vi "Sim Configurations.vi"(8 "error constant":errorcluster, 10 "Base Station":T4, 11 "Cluster in":T1) -> (0 "error constant":errorcluster, 3 "Cluster out":T1)   [LabVIEW 2021]
uses:
  APIs/Controls/Base_Station_Emulator.ctl
  IP Simulation/Controls/Enum-TypeDef.ctl
  Save File/Sim_Confi.ctl
panel:
  out "Data Out":T2
  in  "Enum":T3
  in  "SIM_U_Config":T2
  # "IMSI"
  # "TAC"
  # "K Value"
  # "OP Value"
  # "Edit"
  # "Actions"
  # "Phone Number"
  # "Sim Configurations"
  # "ASDFADFAF"
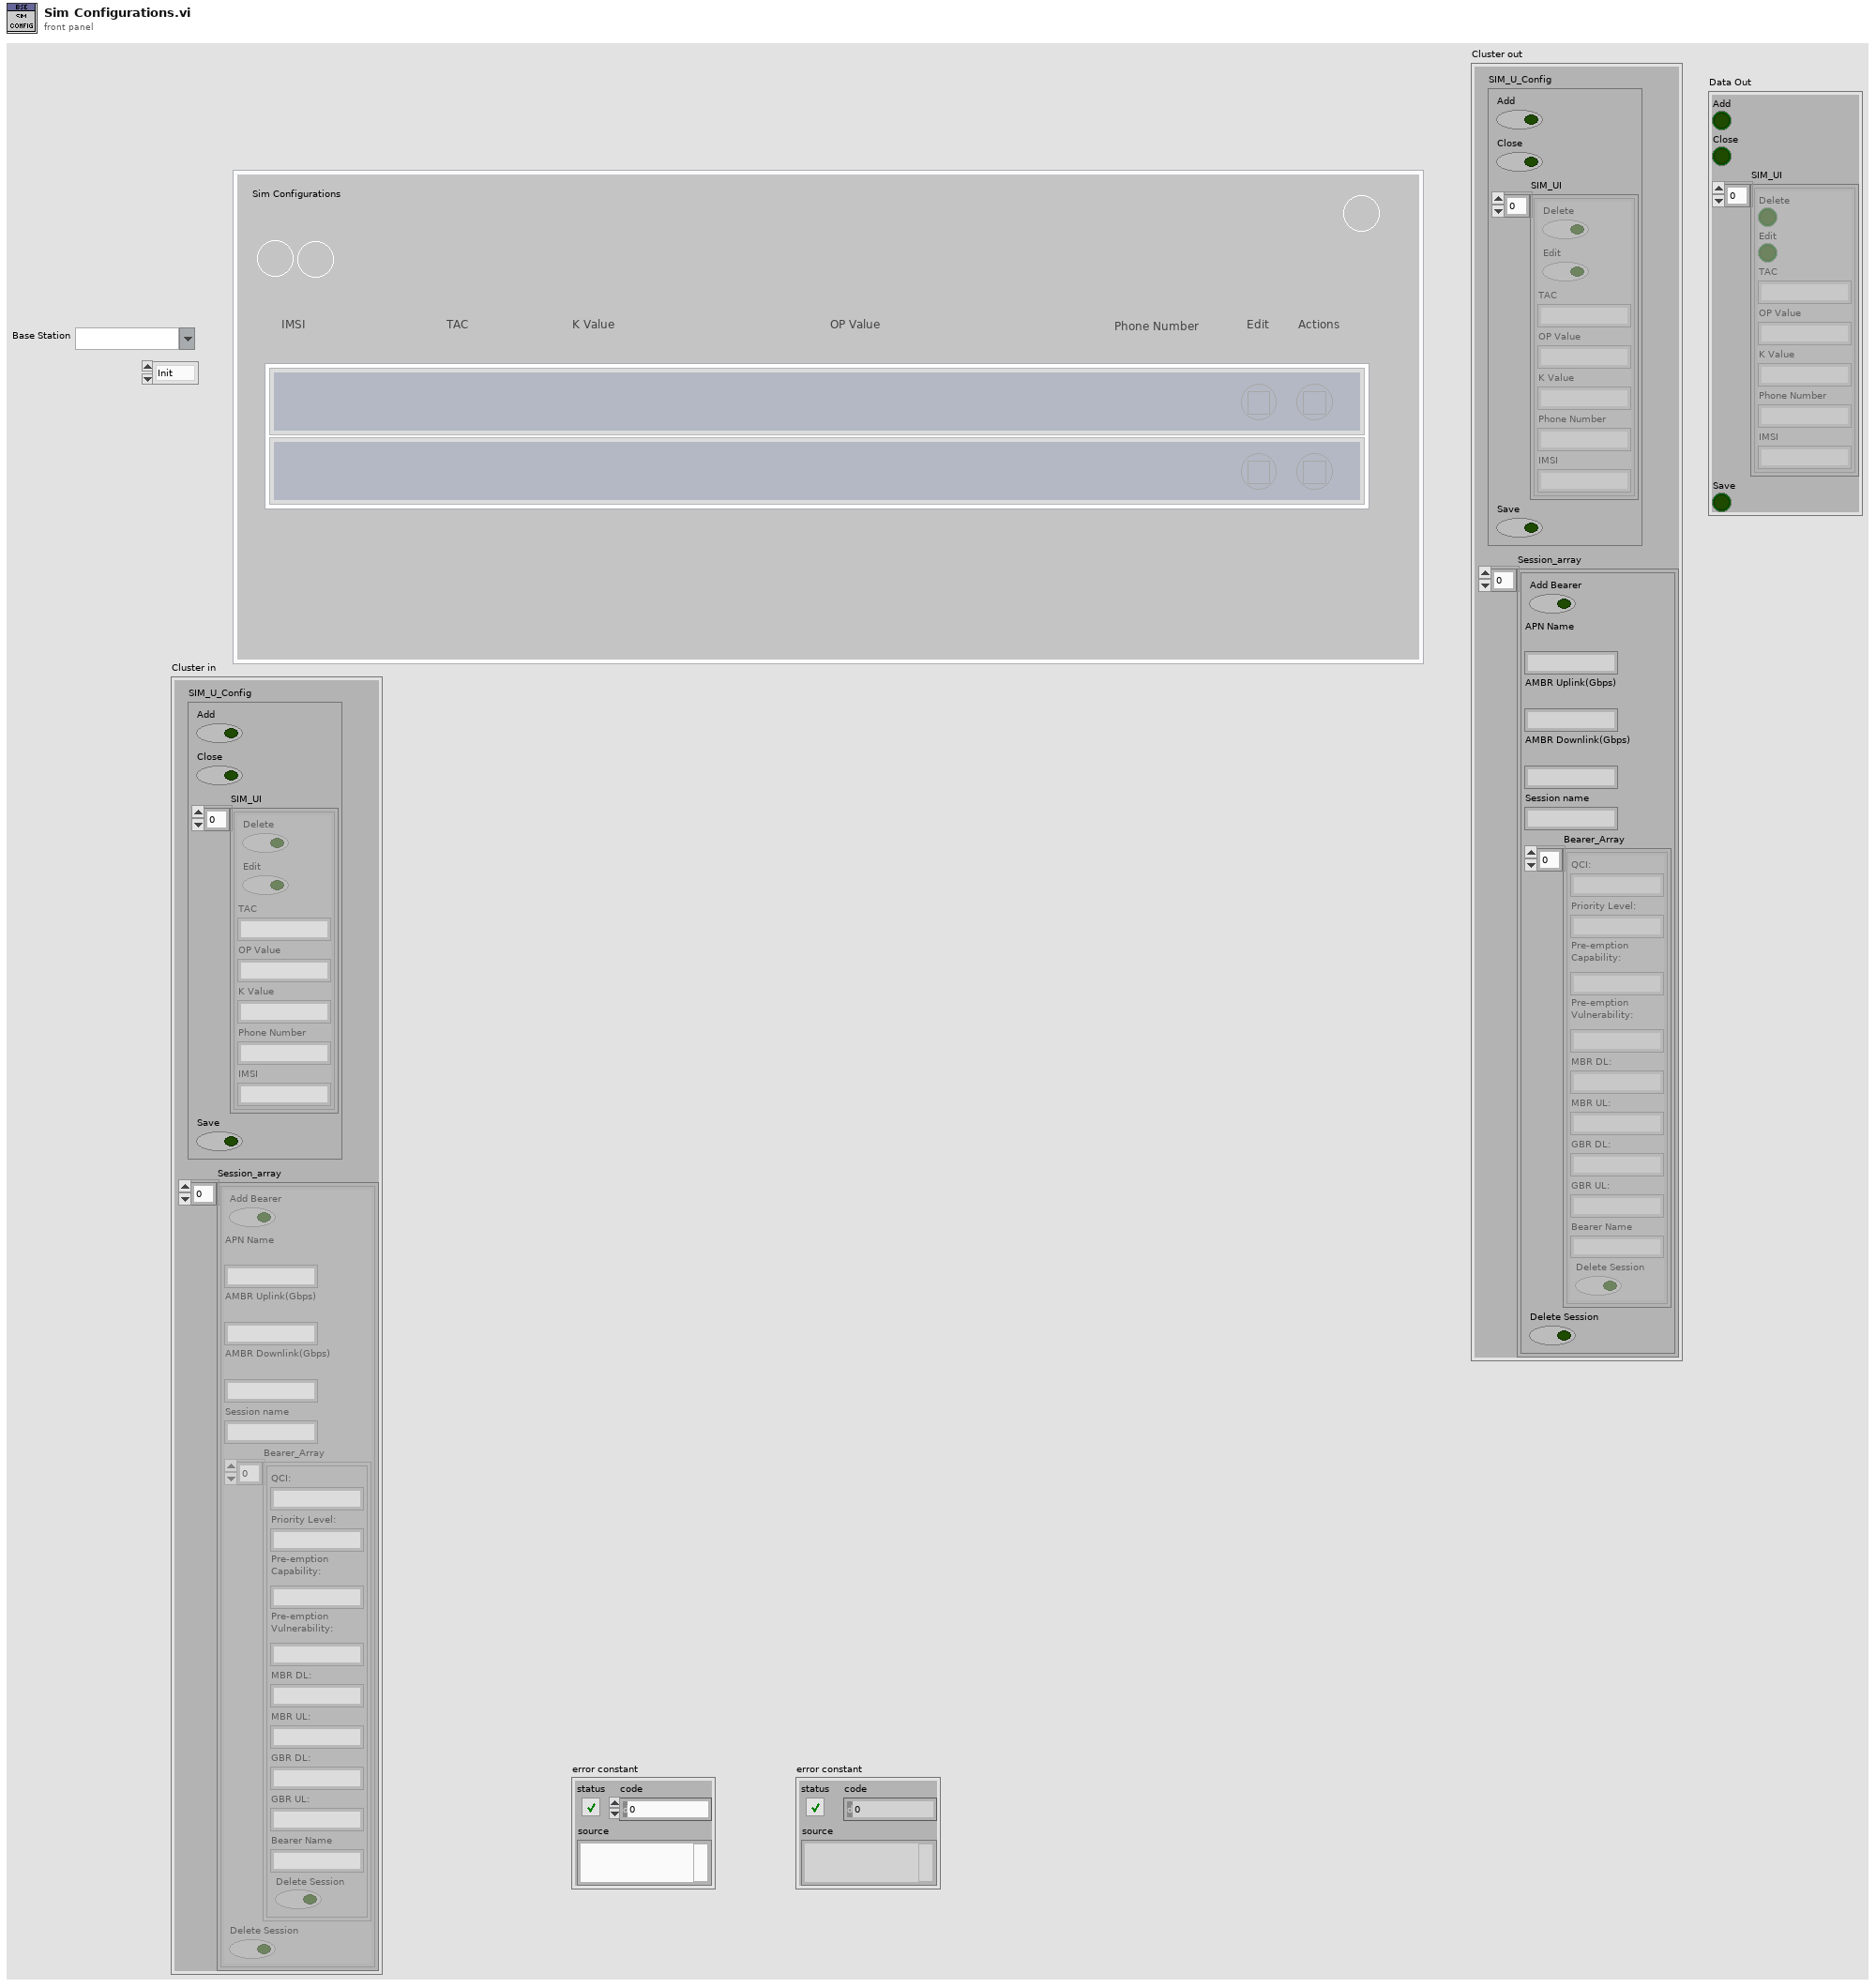
[diagram p1: front panel]
types:
  T1 = typedef "Sim_Confi.ctl" = cluster{"Session_array":cluster{"Add Bearer":bool, "APN Name\n":string, "AMBR Uplink(Gbps)\n":string, "AMBR Downlink(Gbps)\n":string, "Session name":string, "Bearer_Array":cluster{"QCI:":string, "Priority Level:":string, "Pre-emption\nCapability:":string, "Pre-emption\nVulnerability:":string, "MBR DL:":string, "MBR UL:":string, "GBR DL:":string, "GBR UL:":string, "Bearer Name":string, "Delete Session":bool}[], "Delete Session":bool}[], "SIM_U_Config":cluster{"Add":bool, "Close":bool, "SIM_UI":cluster{"Delete":bool, "Edit":bool, "TAC":string, "OP Value":string, "K Value":string, "Phone Number":string, "IMSI":string}[], "Save":bool}}
  T2 = cluster{"Add":bool, "Close":bool, "SIM_UI":cluster{"Delete":bool, "Edit":bool, "TAC":string, "OP Value":string, "K Value":string, "Phone Number":string, "IMSI":string}[], "Save":bool}
  T3 = typedef "Enum-TypeDef.ctl" = enum16{"Init", "poll", "Close"}
  T4 = typedef "Base_Station_Emulator.ctl" = string
  T5 = cluster{"Delete":bool, "Edit":bool, "TAC":string, "OP Value":string, "K Value":string, "Phone Number":string, "IMSI":string}[]
  T6 = cluster{"Add Bearer":bool, "APN Name\n":string, "AMBR Uplink(Gbps)\n":string, "AMBR Downlink(Gbps)\n":string, "Session name":string, "Bearer_Array":cluster{"QCI:":string, "Priority Level:":string, "Pre-emption\nCapability:":string, "Pre-emption\nVulnerability:":string, "MBR DL:":string, "MBR UL:":string, "GBR DL:":string, "GBR UL:":string, "Bearer Name":string, "Delete Session":bool}[], "Delete Session":bool}[]
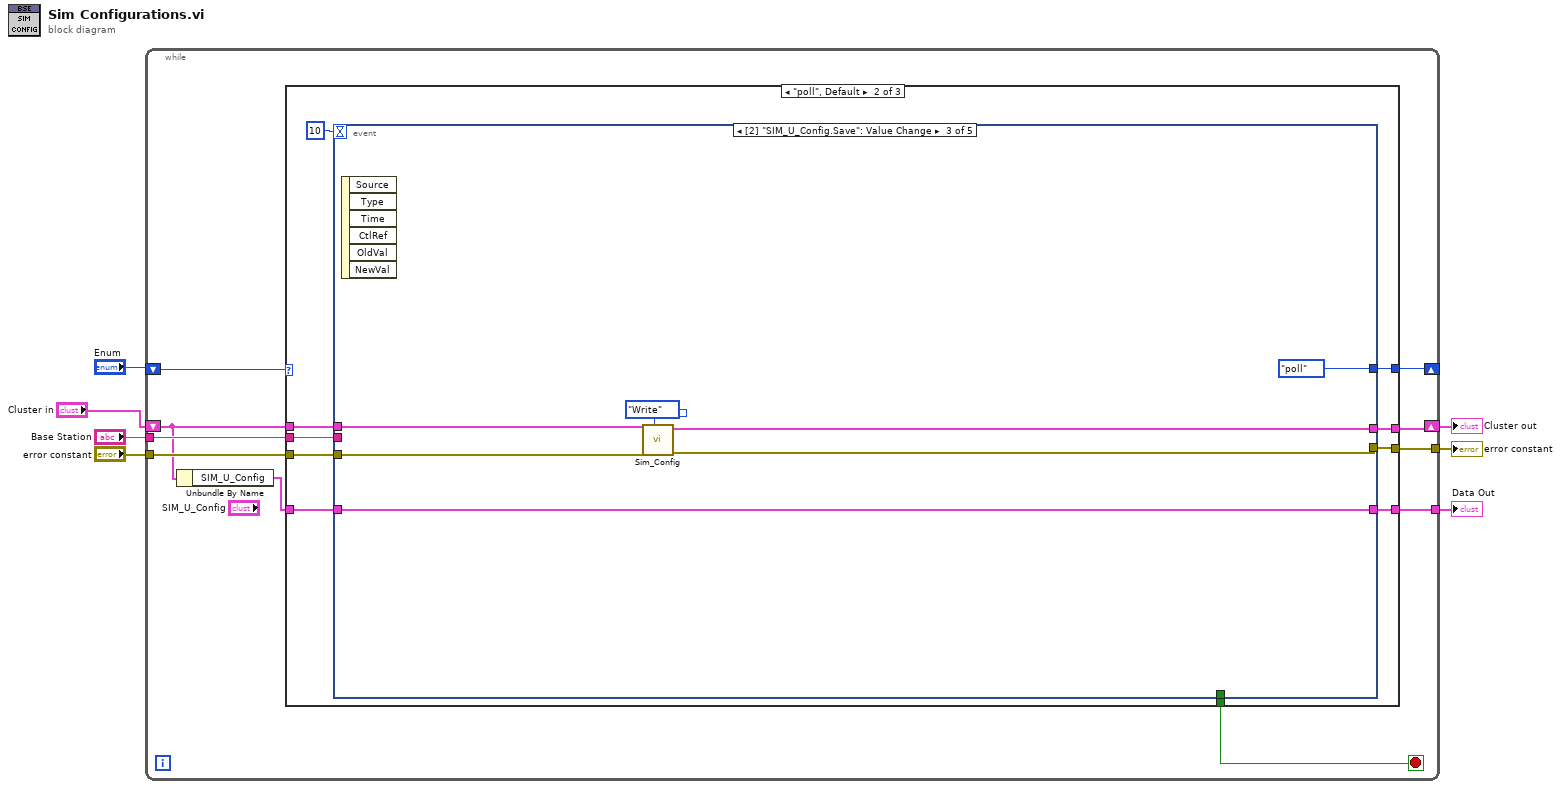
[diagram p0: block diagram]
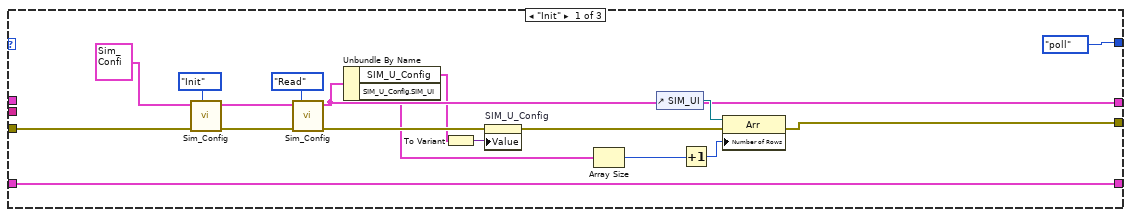
[diagram p2: hidden frame]
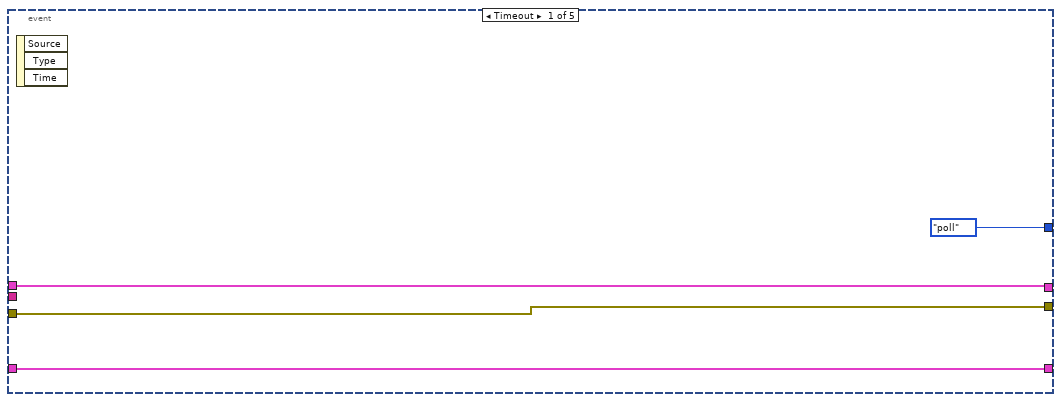
[diagram p3: hidden frame]
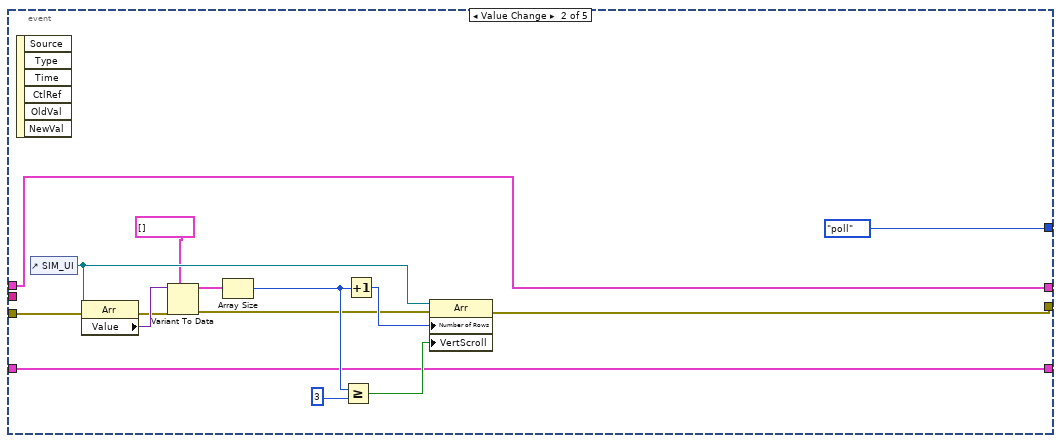
[diagram p4: hidden frame]
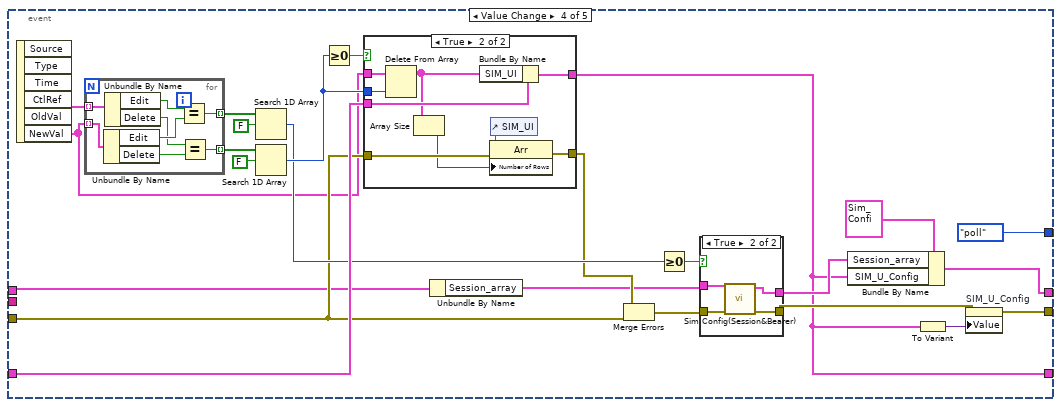
[diagram p5: hidden frame]
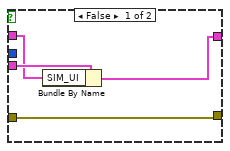
[diagram p6: hidden frame]
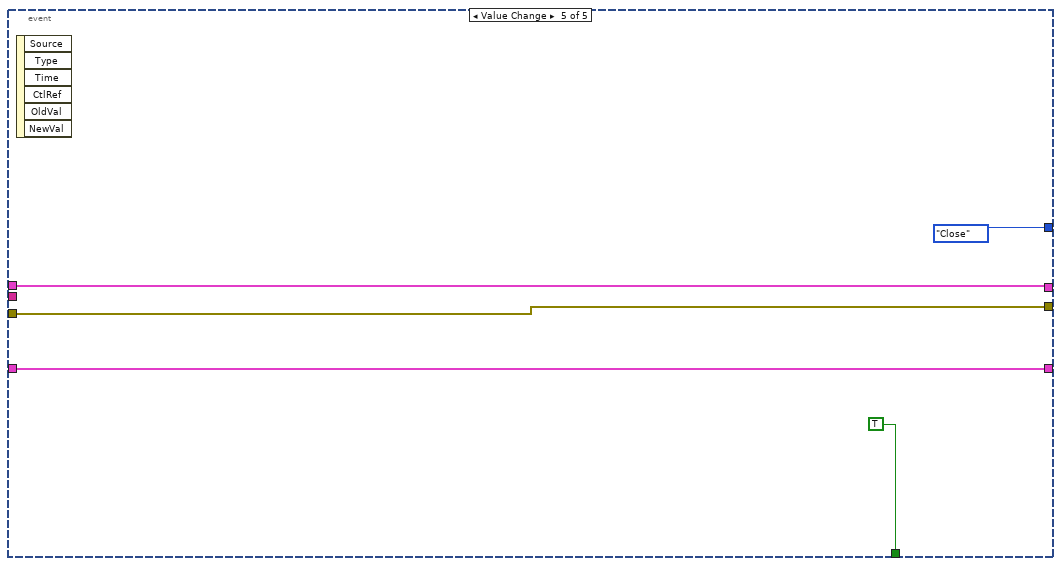
[diagram p8: hidden frame]
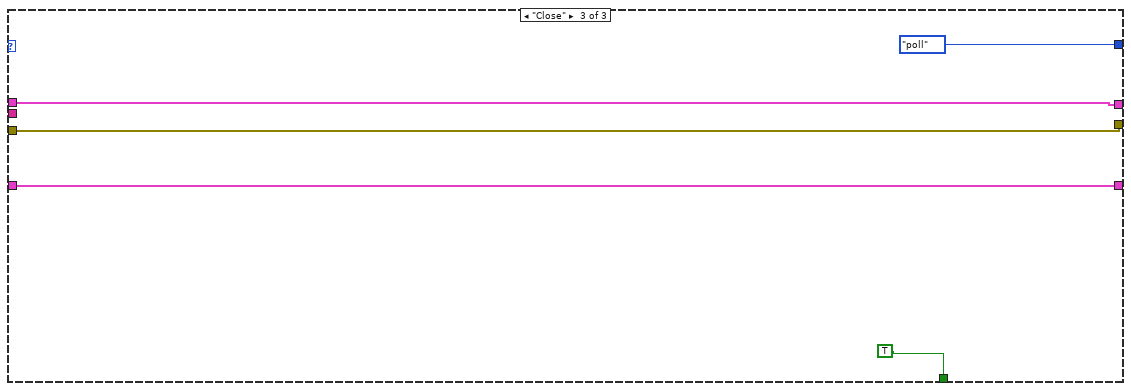
[diagram p9: hidden frame]
diagram:
  n1 = while {
    shift-right: [w15] -> _
    shift-left: "Enum" -> [w16]
    tunnel: "error constant" -> [w14]
    tunnel: [w13] -> w4
    tunnel: "Base Station" -> [w12]
    tunnel: [w11] -> w3
    shift-right: [w10] -> w2
    shift-left: "Cluster in" -> [w9]
    stop <- w17 stop-if-true
    n2 = Unbundle By Name(w9) -> ("SIM_U_Config"=w8:T2)
    n3 = case shown="\"poll\", Default" w16 {
      tunnel: [_ w38 TRUE] -> w17
      tunnel: [Enum-TypeDef."poll" w43 Enum-TypeDef."poll"] -> w15
      tunnel: w14 -> [w21 w45 w131]
      tunnel: [w19 w44 w131] -> w13
      tunnel: w8 -> [w27 w41 w129]
      tunnel: w12 -> [_ w40 _]
      tunnel: [w27 w39 w129] -> w11
      tunnel: [w26 w37 w128] -> w10
      tunnel: w9 -> [_ w36 w128]
      frame "Init" {
        n4 = call "Sim_Config.vi"("Hardware Case Selection"=enum16{"Init", "Read", "Write", "Close"}."Init", "error in (no error)"=w21, 11:T1 {"Session_array"=[{"Add Bearer"=FALSE, "APN Name\n"="", "AMBR Uplink(Gbps)\n"="", "AMBR Downlink(Gbps)\n"="", "Session name"="", "Bearer_Array"=[], "Delete Session"=FALSE}], "SIM_U_Config"={"Add"=FALSE, "Close"=FALSE, "SIM_UI"=[], "Save"=FALSE}}) -> ("error out"=w30:errorcluster, "Cluster"=w22:T1)  [unwired: 7 in]
        n5 = call "Sim_Config.vi"("Hardware Case Selection"=enum16{"Init", "Read", "Write", "Close"}."Read", "error in (no error)"=w30, 11:w22) -> ("error out"=w28:errorcluster, "Cluster"=w26:T1)  [unwired: 7 in]
        n6 = Unbundle By Name(w26) -> ("SIM_U_Config"=w24:T2, "SIM_U_Config.SIM_UI"=w18:T5)
        n7 = To Variant(anything=w24) -> (Variant=w25:variant)
        n8 = property on="SIM_U_Config" class="Clust"(error in=w28, "Value"=w25) -> (error out=w20:errorcluster)  [unwired: 1 in, 1 out]
        n9 = Array Size(array=w18) -> (size(s)=w33:i32)
        n10 = control-ref of="SIM_UI"() -> (w34:refnum<vi>)
        n11 = Increment(x=w33) -> (x+1=w32:i32)
        n12 = property class="Arr"(reference=w34, error in=w20, "Number of Rows"=w32) -> (error out=w19:errorcluster)  [unwired: 1 out]
      }
      frame "poll", Default {
        n13 = event shown="[2] \"SIM_U_Config.Save\": Value Change" {
          selector: _ -> [_ _ _ _ _]
          dyn-events: _ -> [_ _ _ _ _]
          timeout: 10 -> [_ _ _ _ _]
          tunnel: w45 -> [w47 w53 w69 w82 w126]
          tunnel: [w47 w60 w68 w86 w126] -> w44
          tunnel: [Enum-TypeDef."poll" Enum-TypeDef."poll" Enum-TypeDef."poll" Enum-TypeDef."poll" Enum-TypeDef."Close"] -> w43
          tunnel: w40 -> [_ _ _ _ _]
          tunnel: w41 -> [w48 w55 w66 w85 w125]
          tunnel: [w48 w55 w66 w72 w125] -> w39
          tunnel: [_ _ _ _ TRUE] -> w38
          tunnel: [w46 w50 w65 w78 w123] -> w37
          tunnel: w36 -> [w46 w50 w70 w77 w123]
          event Timeout {
            n14 = event-data() -> ()  [unwired: 1 in, 3 out]
          }
          event "SIM_U_Config.Add": Value Change {
            n15 = event-data() -> ()  [unwired: 1 in, 6 out]
            n16 = control-ref of="SIM_UI"() -> (w58:refnum<vi>)
            n17 = property class="Arr"(reference=w58, error in=w53) -> (error out=w52:errorcluster, "Value"=w57:variant)  [unwired: 1 out]
            n18 = Variant To Data(error in=w52, type=T5 [] ("SIM_UI"), Variant=w57) -> (data=w56:T5, error out=w51:errorcluster)
            n19 = Array Size(array=w56) -> (size(s)=w63:i32)
            n20 = Greater Or Equal?(x=w63, y=3) -> (x >= y?=w61:bool)
            n21 = Increment(x=w63) -> (x+1=w59:i32)
            n22 = property class="Arr"(reference=w58, error in=w51, "Number of Rows"=w59, "VertScroll"=w61) -> (error out=w60:errorcluster)  [unwired: 1 out]
          }
          event "SIM_U_Config.Save": Value Change {
            n23 = event-data() -> ()  [unwired: 1 in, 6 out]
            n24 = call "Sim_Config.vi"("Hardware Case Selection"=enum16{"Init", "Read", "Write", "Close"}."Write", "error in (no error)"=w69, 11:w70) -> ("error out"=w68:errorcluster, "Cluster"=w65:T1)  [unwired: 7 in]
          }
          event "SIM_U_Config.SIM_UI": Value Change {
            n25 = event-data() -> ("OldVal"=w92:T5, "NewVal"=w73:T5)  [unwired: 1 in, 4 out]
            n26 = for {
              tunnel: w92 -> [w118] mode=indexing
              tunnel: w73 -> [w122] mode=indexing
              tunnel: [w121] -> w93 mode=indexing
              tunnel: [w115] -> w90 mode=indexing
              n27 = Unbundle By Name(w122) -> ("Edit"=w120:bool, "Delete"=w116:bool)
              n28 = Unbundle By Name(w118) -> ("Edit"=w119:bool, "Delete"=w117:bool)
              n29 = Equal?(x=w119, y=w120) -> (x = y?=w121:bool)
              n30 = Equal?(x=w117, y=w116) -> (x = y?=w115:bool)
            }
            n31 = Search 1D Array(1D array=w93, element=FALSE) -> (index of element=w84:i32)  [unwired: 1 in]
            n32 = Search 1D Array(1D array=w90, element=FALSE) -> (index of element=w88:i32)  [unwired: 1 in]
            n33 = Greater Or Equal To 0?(x=w88) -> (x >= 0?=w89:bool)
            n34 = case shown="True" w89 {
              tunnel: w73 -> [w97 w108]
              tunnel: w88 -> [_ w107]
              tunnel: w85 -> [w98 w106]
              tunnel: [w99 w105] -> w72
              tunnel: w82 -> [w96 w103]
              tunnel: [w96 w100] -> w81
              frame False {
                n35 = Bundle By Name(cluster=w98, "SIM_UI"=w97) -> (w99:T2)
              }
              frame True {
                n36 = Delete From Array(array=w108, index=w107) -> (array with subset deleted=w102:T5)  [unwired: 1 in, 1 out]
                n37 = Array Size(array=w102) -> (size(s)=w101:i32)
                n38 = Bundle By Name(cluster=w106, "SIM_UI"=w102) -> (w105:T2)
                n39 = control-ref of="SIM_UI"() -> (w104:refnum<vi>)
                n40 = property class="Arr"(reference=w104, error in=w103, "Number of Rows"=w101) -> (error out=w100:errorcluster)  [unwired: 1 out]
              }
            }
            n41 = Unbundle By Name(w77) -> ("Session_array"=w79:T6)
            n42 = Merge Errors(w81, w82) -> (w80:errorcluster)
            n43 = Greater Or Equal To 0?(x=w84) -> (x >= 0?=w83:bool)
            n44 = case shown="True" w83 {
              tunnel: w80 -> [w110 w114]
              tunnel: [w110 w113] -> w76
              tunnel: w79 -> [w109 w111]
              tunnel: [w109 w112] -> w74
              frame False {
              }
              frame True {
                n45 = call "Sim Config(Session&Bearer).vi"("error constant"=w114, "Session_array"=w111) -> ("error constant"=w113:errorcluster, "Session_array 2"=w112:T6)  [unwired: 8 in]
              }
            }
            n46 = Bundle By Name(cluster=T1 {"Session_array"=[{"Add Bearer"=FALSE, "APN Name\n"="", "AMBR Uplink(Gbps)\n"="", "AMBR Downlink(Gbps)\n"="", "Session name"="", "Bearer_Array"=[], "Delete Session"=FALSE}], "SIM_U_Config"={"Add"=FALSE, "Close"=FALSE, "SIM_UI"=[], "Save"=FALSE}} ("Cluster"), "Session_array"=w74, "SIM_U_Config"=w72) -> (w78:T1)
            n47 = To Variant(anything=w72) -> (Variant=w87:variant)
            n48 = property on="SIM_U_Config" class="Clust"(error in=w76, "Value"=w87) -> (error out=w86:errorcluster)  [unwired: 1 in, 1 out]
          }
          event "SIM_U_Config.Close": Value Change {
            n49 = event-data() -> ()  [unwired: 1 in, 6 out]
          }
        }
      }
      frame "Close" {
      }
    }
  }
  "error constant" <- w4
  "Data Out" <- w3
  "Cluster out" <- w2
